vi "SetUSB5GlobalSoftTrig.vi"(8 "错误输入（无错误）":errorcluster, 11 "DevIndex":i32) -> (0 "错误输出":errorcluster, 3 "DevIndex Out":i32)   [LabVIEW 2020]
uses:
  lib/x64/USB5000.dll
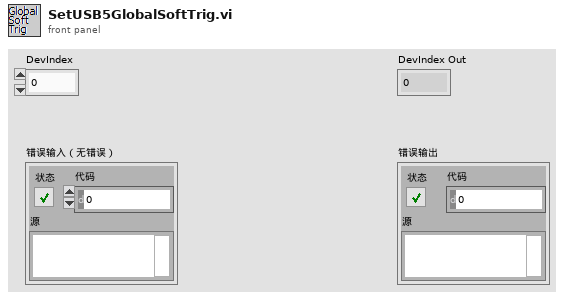
[diagram p1: front panel]
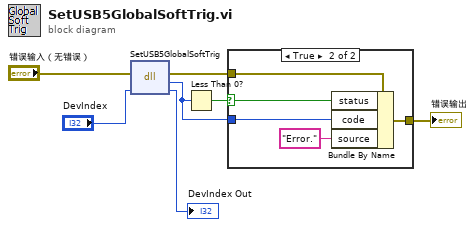
[diagram p0: block diagram]
diagram:
  n1 = dll-call lib="C:/Users/phosense/Downloads/USB-5000/usb5000_labview_cv/lib/x64/USB5000.dll" fn="SetUSB5GlobalSoftTrig"(error in="错误输入（无错误）", "DevIndex"="DevIndex") -> (error out=w3:errorcluster, "返回类型"=w2:i32, "DevIndex"=→"DevIndex Out":i32)  [unwired: 2 in, 1 out]
  n2 = Less Than 0?(x=w2) -> (x < 0?=w4:bool)
  n3 = case shown="True" w4 {
    selector: w4 -> [_ w9]
    tunnel: [w8 w11] -> w1
    tunnel: w2 -> [_ w13]
    tunnel: w3 -> [w8 w10]
    frame False {
    }
    frame True {
      n4 = Bundle By Name(cluster=w10, "status"=w9, "code"=w13, "source"="Error." ("error message (\"\")")) -> (w11:errorcluster)
    }
  }
  "错误输出" <- w1
